vi "mainog_write out of loop.vi"() -> ()   [LabVIEW 2014]
uses:
  <vilib>/Instr/_visa.llb/VISA Configure Serial Port (Instr).vi
panel:
  in  "Write Pressure Values 2":bool
  out "12bit DAC signal sent 2":string
  in  "Desired Pressures 2":dbl[](array[numeric])
  in  "Keep Data?":bool
  in  "filepath:":path
  out "Pressure Plot":i32[](graph)
  out "mbar":string[](array[string])
  out "status":bool
  out "error out":errorcluster
  in  "error in":errorcluster
  in  "stop":bool
  # "Arduino LabVIEW - Serial Read and Write"
  # "Measured Pressures"
  # "Desired pressures must be expressed in volts (0-5)"
  # "Channel 1"
  # "Channel 2"
  # "Channel 1"
  # "Channel 3"
  # "Channel 2"
  # "Channel 4"
  # "Channel 3"
  # "Channel 4"
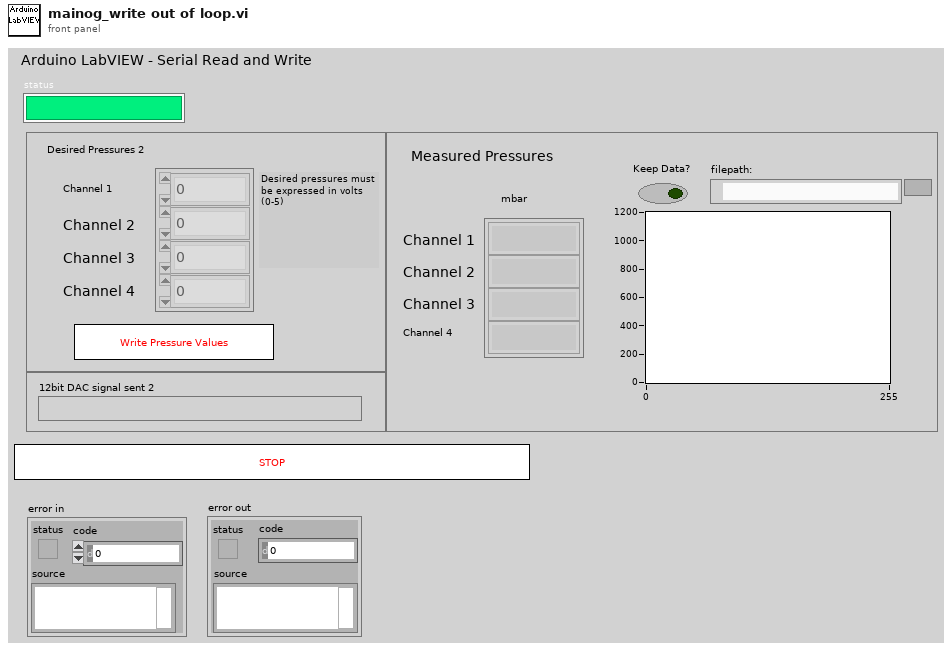
[diagram p1: front panel]
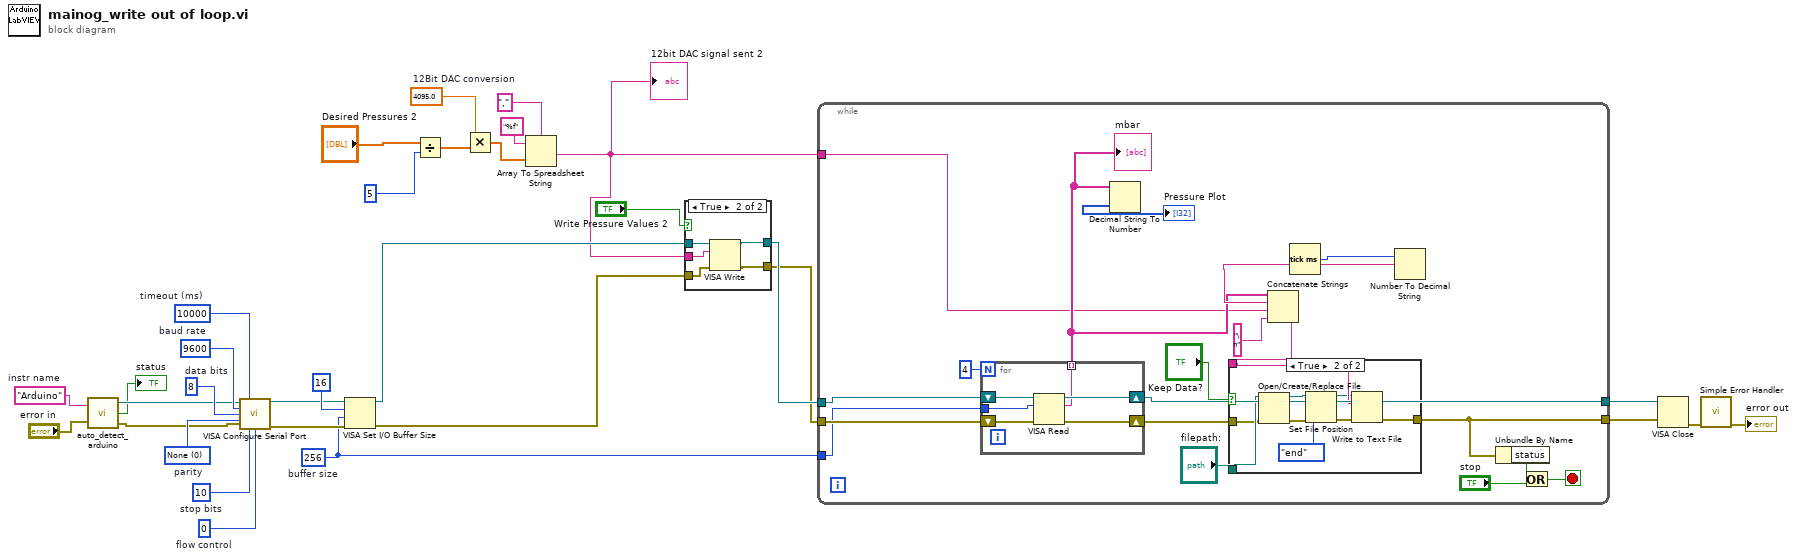
[diagram p0: block diagram]
diagram:
  w8 = 4095.0  # 12Bit DAC conversion
  w23 = "Arduino"  # instr name
  w19 = u32 256  # buffer size
  w30 = u16 0  # flow control
  w29 = u16 10  # stop bits
  w28 = u16 0 items=["None", "Odd", "Even", "Mark", "Space"]  # parity
  w27 = u16 8  # data bits
  w26 = u32 9600  # baud rate
  w31 = u32 10000  # timeout (ms)
  n1 = call "auto_detect_arduino.vi"("instr name"=w23, "error in"="error in") -> ("VISA resource name"=w25:refnum<visa-resource-name>, "status"=→"status":bool, "error out"=w24:errorcluster)
  n2 = call-poly "VISA Configure Serial Port"("VISA resource name"=w25, "timeout (10sec)"=w31, "baud rate (9600)"=w26, "data bits (8)"=w27, "parity (0:none)"=w28, "error in (no error)"=w24, "stop bits (10: 1 bit)"=w29, "flow control (0:none)"=w30) -> ("VISA resource name out"=w21:refnum<visa-resource-name>, "error out"=w20:errorcluster)  [unwired: 6 in]
  n3 = VISA Set I/O Buffer Size(VISA resource name=w21, mask (16)=u16 16 ("I/O Receive\nBuffer mask"), size (4096)=w19, error in (no error)=w20) -> (VISA resource name out=w5:refnum<visa-resource-name>, error out=w3:errorcluster)
  n4 = Divide(x="Desired Pressures 2", y=5) -> (x/y=w10:dbl[])
  n5 = Multiply(x=w8, y=w10) -> (x*y=w9:dbl[])
  n6 = Array To Spreadsheet String(delimiter (Tab)=",", array=w9, 3:"%f" ("format string")) -> (spreadsheet string=w1:string)
  "12bit DAC signal sent 2" <- w1
  n7 = case shown="True" "Write Pressure Values 2" {
    tunnel: [w34 w39] -> w4
    tunnel: [w33 w38] -> w2
    tunnel: w5 -> [w34 w37]
    tunnel: w3 -> [w33 w36]
    tunnel: w1 -> [_ w35]
    frame False {
    }
    frame True {
      n8 = VISA Write(VISA resource name=w37, write buffer=w35, error in (no error)=w36) -> (VISA resource name out=w39:refnum<visa-resource-name>, error out=w38:errorcluster)  [unwired: 1 out]
    }
  }
  n9 = while {
    tunnel: [w56] -> w32
    tunnel: w19 -> [w42]
    tunnel: [w51] -> w14
    tunnel: w4 -> [w44]
    tunnel: w2 -> [w43]
    tunnel: w1 -> [w40]
    stop <- w57 stop-if-true
    n10 = for {
      N: 4 -> [_]
      tunnel: [w70] -> w45 mode=indexing
      shift-right: [w73] -> w56
      shift-left: w44 -> [w72]
      shift-right: [w74] -> w52
      shift-left: w43 -> [w71]
      tunnel: w42 -> [w69]
      n11 = VISA Read(VISA resource name=w72, byte count=w69, error in (no error)=w71) -> (VISA resource name out=w73:refnum<visa-resource-name>, read buffer=w70:string, error out=w74:errorcluster)  [unwired: 1 out]
    }
    "mbar" <- w45
    n12 = Decimal String To Number(string=w45) -> (number=→"Pressure Plot":i32[])  [unwired: 2 in, 1 out]
    n13 = Tick Count (ms)() -> (millisecond timer value=w46:u32)
    n14 = Number To Decimal String(number=w46) -> (decimal integer string=w47:string)  [unwired: 1 in]
    n15 = Concatenate Strings(w45, w47, w40, "\n" ("string")) -> (w48:string)
    n16 = case shown="True" "Keep Data?" {
      tunnel: w48 -> [_ w68]
      tunnel: "filepath:" -> [_ w67]
      tunnel: w52 -> [w59 w66]
      tunnel: [w59 w61] -> w51
      frame False {
      }
      frame True {
        n17 = Open/Create/Replace File(file path (use dialog)=w67, error in=w66) -> (refnum out=w64:refnum<file>, error out=w65:errorcluster)  [unwired: 4 in, 1 out]
        n18 = Set File Position(refnum=w64, from (0:start)=enum16{"start", "end", "current"}."end", error in=w65) -> (refnum out=w63:refnum<file>, error out=w62:errorcluster)  [unwired: 1 in]
        n19 = Write to Text File(file (use dialog)=w63, text=w68, error in=w62) -> (error out=w61:errorcluster)  [unwired: 1 in, 2 out]
      }
    }
    n20 = Unbundle By Name(w51) -> ("status"=w50:bool)
    n21 = Or(x=w50, y="stop") -> (x .or. y?=w57:bool)
  }
  n22 = VISA Close(VISA resource name=w32, error in (no error)=w14) -> (error out=w17:errorcluster)
  n23 = call <vilib>:"Simple Error Handler.vi"("error in (no error)"=w17) -> ("error out"=→"error out":errorcluster)  [unwired: 4 in, 4 out]
